vi "Take a Measurement.vi"(0 "Register Buses":T1[](array[typedef]), 11 "error in":errorcluster) -> (4 "Register Buses (out)":T1[](array[typedef]), 8 "measurement values":u16[](array[numeric]), 10 "measurement valid":bool, 15 "error out":errorcluster)   [LabVIEW 2014, in "ni579x Synchronization v2 Host.lvlib"]
uses:
  <instrlib>/ni579x/Synchronization/v2/Host/ni579x Synchronization v2 Host.lvlib
  <instrlib>/_niInstr/Register Bus/v0/Host/Public/Register Bus Session.ctl
  <instrlib>/_niInstr/Register Bus/v0/Host/Private/Session Data.ctl
  <instrlib>/ni579x/Synchronization/v2/Shared/ni579x Synchronization Register Addresses.ctl
  <instrlib>/ni579x/Config/v2/Shared/Types/ni579x Register Bus Subsystem ID.ctl
  <instrlib>/_niInstr/Register Bus/v0/Host/Public/Register Write.ctl
  <instrlib>/_niInstr/Register Bus/v0/Host/Public/Register Read Request.ctl
  <instrlib>/ni579x/Config/v2/Shared/ni579x Config v2 Shared.lvlib
  <instrlib>/_niInstr/Register Bus/v0/Host/niInstr Register Bus v0 Host.lvlib
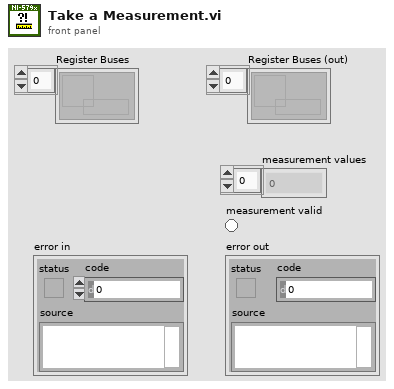
[diagram p1: front panel]
types:
  T1 = typedef "niInstr Register Bus v0 Host.lvlib/Register Bus Session.ctl" = refnum<queue>
  T2 = typedef "niInstr Register Bus v0 Host.lvlib/Register Read Request.ctl" = cluster{"subsystem":u8, "address":u16}
  T3 = typedef "niInstr Register Bus v0 Host.lvlib/Register Write.ctl" = cluster{"subsystem":u8, "address":u16, "data":u32}
  T4 = typedef "ni579x Config v2 Shared.lvlib/ni579x Register Bus Subsystem ID.ctl" = u8
  T5 = typedef "ni579x Synchronization Register Addresses.ctl" = enum16{"Signature", "Current Version", "Oldest Compatible Version", "Scratch Register", "sync.master", "sync.meas.enable", "sync.meas.ready", "sync.meas.arm", "sync.meas.valid", "sync.meas.value", "sync.cptr.adjust", "sync.cptr.period", "sync.meas.oversample factor"}
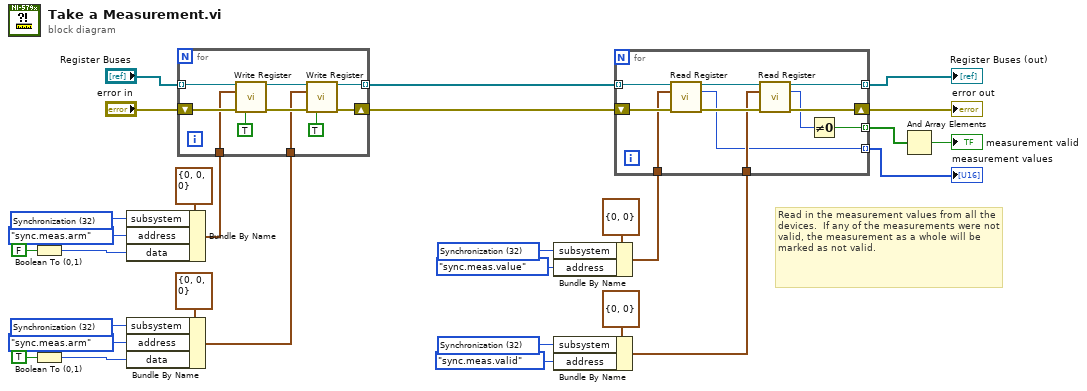
[diagram p0: block diagram]
diagram:
  w14 = T4 32 items=["FAM Register Operation"=0, "User Command"=16, "Synchronization"=32] ("Subsystem ID")
  w16 = T4 32 items=["FAM Register Operation"=0, "User Command"=16, "Synchronization"=32] ("Subsystem ID")
  w20 = T4 32 items=["FAM Register Operation"=0, "User Command"=16, "Synchronization"=32] ("Subsystem ID")
  w25 = T4 32 items=["FAM Register Operation"=0, "User Command"=16, "Synchronization"=32] ("Subsystem ID")
  # "Read in the measurement values from all the devices.  If any of the measurements were not valid, the measurement as a whole will be marked as not valid."
  n1 = Boolean To (0,1)(Boolean=FALSE ("sync.Master")) -> (0, 1=w27:i16)
  n2 = Boolean To (0,1)(Boolean=TRUE ("sync.Master")) -> (0, 1=w18:i16)
  n3 = Bundle By Name(cluster=T3 {"subsystem"=0, "address"=0, "data"=0} ("register write"), "subsystem"=w25, "address"=ni579x_Synchronization_Register_Addresses."sync.meas.arm" ("Synchronization Registers"), "data"=w27) -> (w28:T3)
  n4 = Bundle By Name(cluster=T3 {"subsystem"=0, "address"=0, "data"=0} ("register write"), "subsystem"=w20, "address"=ni579x_Synchronization_Register_Addresses."sync.meas.arm" ("Synchronization Registers"), "data"=w18) -> (w5:T3)
  n5 = for {
    tunnel: "Register Buses" -> [w39] mode=indexing
    tunnel: w28 -> [w37]
    tunnel: [w34] -> w15 mode=indexing
    shift-right: [w33] -> w22
    shift-left: "error in" -> [w38]
    tunnel: w5 -> [w31]
    n6 = call <instrlib>:"Write Register.vi"("session in"=w39, "register write"=w37, "error in"=w38, "wait until committed"=TRUE) -> ("session out"=w35:T1, "error out"=w32:errorcluster)  [unwired: 10 in]
    n7 = call <instrlib>:"Write Register.vi"("session in"=w35, "register write"=w31, "error in"=w32, "wait until committed"=TRUE) -> ("session out"=w34:T1, "error out"=w33:errorcluster)  [unwired: 10 in]
  }
  n8 = Bundle By Name(cluster=T2 {"subsystem"=0, "address"=0} ("register read request"), "subsystem"=w16, "address"=ni579x_Synchronization_Register_Addresses."sync.meas.value" ("Synchronization Registers")) -> (w12:T2)
  n9 = Bundle By Name(cluster=T2 {"subsystem"=0, "address"=0} ("register read request"), "subsystem"=w14, "address"=ni579x_Synchronization_Register_Addresses."sync.meas.valid" ("Synchronization Registers")) -> (w11:T2)
  n10 = for {
    tunnel: w15 -> [w48] mode=indexing
    tunnel: [w46] -> w6 mode=indexing
    shift-right: [w45] -> w7
    shift-left: w22 -> [w50]
    tunnel: w12 -> [w44]
    tunnel: w11 -> [w43]
    tunnel: [w41] -> w8 mode=indexing
    tunnel: [w40] -> w10 mode=indexing
    n11 = call <instrlib>:"Read Register.vi"("session in"=w48, "register read request"=w44, "error in"=w50) -> ("session out"=w47:T1, "data"=w41:u32, "error out"=w49:errorcluster)  [unwired: 10 in]
    n12 = call <instrlib>:"Read Register.vi"("session in"=w47, "register read request"=w43, "error in"=w49) -> ("session out"=w46:T1, "data"=w42:u32, "error out"=w45:errorcluster)  [unwired: 10 in]
    n13 = Not Equal To 0?(x=w42) -> (x != 0?=w40:bool)
  }
  "error out" <- w7
  "measurement values" <- w8
  "Register Buses (out)" <- w6
  n14 = And Array Elements(Boolean array=w10) -> (logical AND=→"measurement valid":bool)
